vi "Multi Enqueue.vi"(6 "Enqueue Mode":T1, 8 "error in (no error)":errorcluster, 10 "Array of Queue Data":T2[](array[typedef]), 11 "Messaging in":refnum<class "Messaging.lvclass">) -> (0 "error out":errorcluster, 3 "Messaging out":refnum<class "Messaging.lvclass">)   [LabVIEW 2023, in "MessagingModule.lvlib" / "Messaging.lvclass"]
uses:
  Messaging.lvclass
  Messaging.lvclass/Messaging.ctl
  Msg/Msg.Data.ctl
  MessagingModule.lvlib
  Msg/Msg.Q.EnqueueMode.ctl
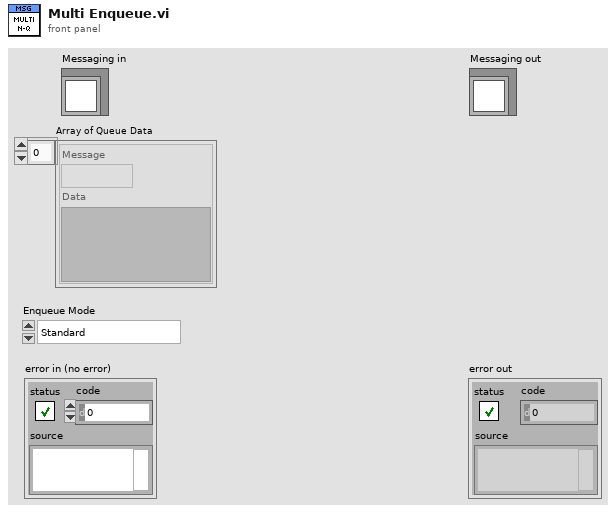
[diagram p1: front panel]
types:
  T1 = typedef "MessagingModule.lvlib/Msg.Q.EnqueueMode.ctl" = enum16{"Standard", "Lossy"}
  T2 = typedef "MessagingModule.lvlib/Msg.Data.ctl" = cluster{"Message":string, "Data":variant}
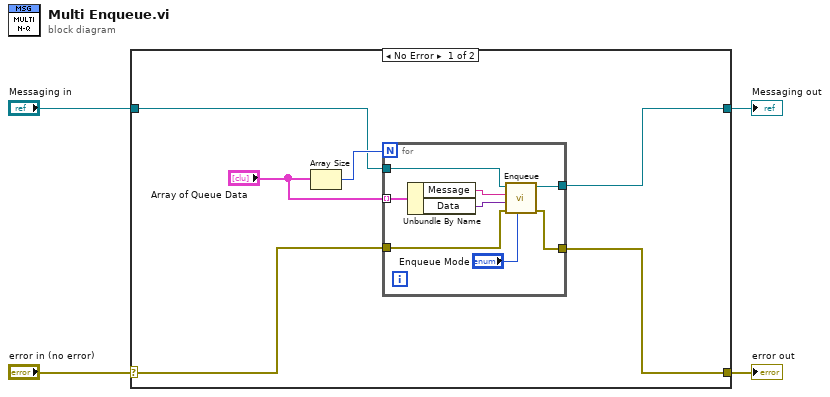
[diagram p0: block diagram]
diagram:
  n1 = case shown="No Error" "error in (no error)" {
    selector: "error in (no error)" -> [w8 w20]
    tunnel: [w7 w20] -> w3
    tunnel: [w5 w19] -> w1
    tunnel: "Messaging in" -> [w6 w19]
    frame No Error {
      n2 = Array Size(array="Array of Queue Data") -> (size(s)=w10:i32)
      n3 = for {
        N: w10 -> [_]
        tunnel: "Array of Queue Data" -> [w18] mode=indexing
        tunnel: w8 -> [w15]
        tunnel: [w14] -> w7
        tunnel: w6 -> [w12]
        tunnel: [w11] -> w5
        n4 = Unbundle By Name(w18) -> ("Message"=w17:string, "Data"=w16:variant)
        n5 = call "Enqueue.vi"("Enqueue Mode"="Enqueue Mode", "error in (no error)"=w15, "Data"=w16, "Message"=w17, "Messaging in"=w12) -> ("error out"=w14:errorcluster, "Messaging out"=w11:refnum<class "Messaging.lvclass">)  [unwired: 5 in]
      }
    }
    frame Error {
    }
  }
  "error out" <- w3
  "Messaging out" <- w1
